vi "UDT_LoggingModule_sendCloseLog.vi"() -> (3 "Unit Test Framework Results":T1)   [LabVIEW 2017]
doc: "Use this template to create a user-defined test VI. Define your test requirements and wire the results to the <b>Result (Test)</b> control. Do not modify the <b>Unit Test Framework Results</b> indicator."
uses:
  <vilib>/utf/common/utf_test_result_troll.ctl
  <vilib>/utf/common/utf_test_result.ctl
  <vilib>/utf/common/utf_test_result_failure.ctl
  <vilib>/utf/common/utf_test_comparison_operators.ctl
  <vilib>/utf/common/utf_vi_tag.ctl
  RT/loggingModule/Queue/TypeDefs/queueFGVState.ctl
  RT/loggingModule/loggingModule.lvlib
  <vilib>/Control Software Solutions Ltd/UTF Helper/Unit Test Helper.lvlib
  <vilib>/utf/NI_UnitTestFramework.lvlib
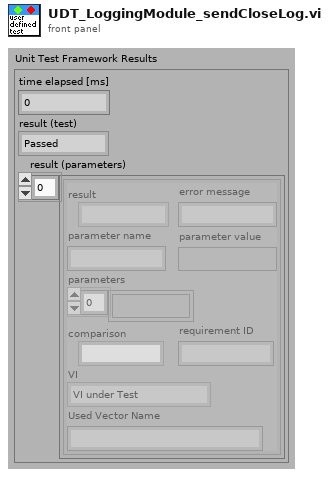
[diagram p1: front panel]
types:
  T1 = typedef "NI_UnitTestFramework.lvlib/utf_test_result_troll.ctl" = cluster{"time elapsed [ms]":u32, "result (test)":T2, "result (parameters)":T3[]}
  T2 = typedef "NI_UnitTestFramework.lvlib/utf_test_result.ctl" = enum16{"Passed", "Failed", "Error", "Skipped", "Not Processed"}
  T3 = typedef "NI_UnitTestFramework.lvlib/utf_test_result_failure.ctl" = cluster{"result":T2, "error message":string, "parameter name":string, "parameter value":variant, "parameters":variant[], "comparison":T4, "requirement ID":string, "VI":T5, "Used Vector Name":string}
  T4 = typedef "NI_UnitTestFramework.lvlib/utf_test_comparison_operators.ctl" = enum16{"=", "!=", ">", ">=", "<", "<=", "range", "symmetric tolerance", "asymmetric tolerance", "string contains", "string not contain", "array size", "string length", "array range", "by element", "array range (limit array)", "user-defined", "array contains", "array not contain", "vector length", "= (elm)", "!= (elm)", "= (case insensitive)", "!= (case insensitive)"}
  T5 = typedef "NI_UnitTestFramework.lvlib/utf_vi_tag.ctl" = enum16{"Setup VI", "VI under Test", "Teardown VI"}
  T6 = typedef "loggingModule.lvlib/queueFGVState.ctl" = enum16{"obtain", "enqueue low priority", "enqueue high priority", "dequeue", "release"}
  T7 = typedef "loggingModule.lvlib/message.ctl" = cluster{"calling module":string, "message":string, "data":variant}
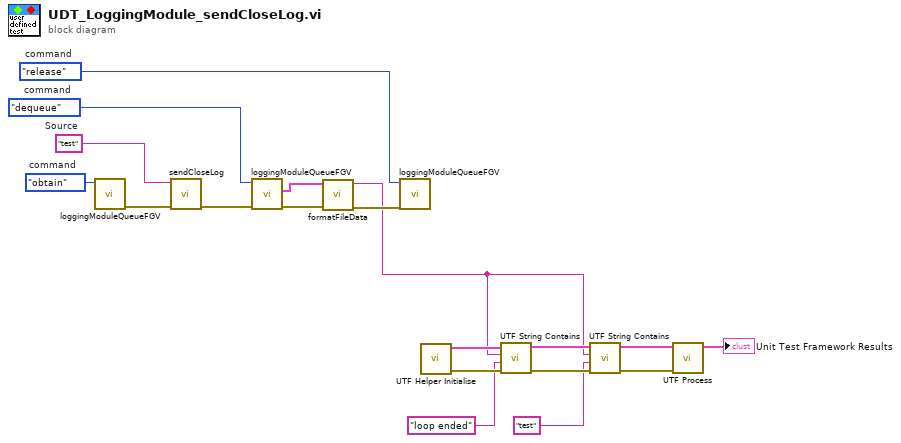
[diagram p0: block diagram]
diagram:
  w14 = queueFGVState."release"  # command
  w15 = queueFGVState."dequeue"  # command
  w17 = "test"  # Source
  w19 = queueFGVState."obtain"  # command
  n1 = call "loggingModuleQueueFGV.vi"("command"=w19) -> ("error out"=w18:errorcluster)  [unwired: 9 in, 1 out]
  n2 = call "sendCloseLog.vi"("error in (no error)"=w18, "Source"=w17) -> ("error out"=w16:errorcluster)  [unwired: 9 in]
  n3 = call "loggingModuleQueueFGV.vi"("error in (no error)"=w16, "command"=w15) -> ("error out"=w6:errorcluster, "message out"=w4:T7)  [unwired: 8 in]
  n4 = call "formatFileData.vi"("error in (no error)"=w6, "message out"=w4) -> ("error out"=w5:errorcluster, "LogData"=w3:string)  [unwired: 8 in]
  n5 = call "loggingModuleQueueFGV.vi"("error in (no error)"=w5, "command"=w14) -> ()  [unwired: 8 in, 2 out]
  n6 = call <vilib>:"UTF Helper Initialise.vi"() -> ("error out"=w7:errorcluster, "results array"=w8:T3[])  [unwired: 10 in]
  n7 = call <vilib>:"UTF String Contains.vi"("error in (no error)"=w7, "Test Value"="loop ended", "Input"=w3, "Input Results"=w8) -> ("error out"=w9:errorcluster, "Output Results"=w10:T3[])  [unwired: 6 in]
  n8 = call <vilib>:"UTF String Contains.vi"("error in (no error)"=w9, "Test Value"="test", "Input"=w3, "Input Results"=w10) -> ("error out"=w12:errorcluster, "Output Results"=w11:T3[])  [unwired: 6 in]
  n9 = call <vilib>:"UTF Process.vi"("error in (no error)"=w12, "results array"=w11) -> ("Unit Test Framework Results"=→"Unit Test Framework Results":T1)  [unwired: 9 in]
